vi "G1DUArr.vi"() -> (0 "1D UArr":u64[](array[numeric]))   [LabVIEW 2023]
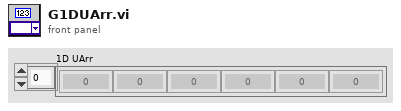
[diagram p1: front panel]
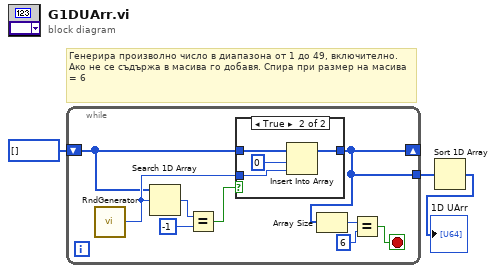
[diagram p0: block diagram]
diagram:
  # "Генерира произволно число в диапазона от 1 до 49, включително.\nАко не се съдържа в масива го добавя. Спира при размер на масива = 6"
  n1 = while {
    shift-right: [w4] -> _
    shift-left: u64[] [] -> [w5]
    tunnel: [w4] -> w2
    stop <- w7 stop-if-true
    n2 = call "RndGenerator.vi"() -> ("Double digit"=w6:u64)  [unwired: 10 in, 1 out]
    n3 = Search 1D Array(1D array=w5, element=w6) -> (index of element=w12:i32)  [unwired: 1 in]
    n4 = Equal?(x=w12, y=-1) -> (x = y?=w10:bool)
    n5 = case shown="True" w10 {
      tunnel: [w13 w14] -> w4
      tunnel: w6 -> [_ w16]
      tunnel: w5 -> [w13 w15]
      frame False {
      }
      frame True {
        n6 = Insert Into Array(array=w15, index=0, new element=w16) -> (w14:u64[])
      }
    }
    n7 = Array Size(array=w4) -> (size(s)=w9:i32)
    n8 = Equal?(x=w9, y=6) -> (x = y?=w7:bool)
  }
  n9 = Sort 1D Array(array=w2) -> (sorted array=→"1D UArr":u64[])
